vi "Start Sync.vi"(8 "error in (no error)":errorcluster, 11 "gRPC service in":refnum<class "OOBgRPCService.lvclass">) -> (0 "error out":errorcluster, 3 "gRPC service out":refnum<class "OOBgRPCService.lvclass">)   [LabVIEW 2025, in "OOB gRPC Server.lvlib" / "OOBgRPCService.lvclass"]
uses:
  OOBgRPCService.lvclass
  OOBgRPCService.lvclass/OOBgRPCService.ctl
  RPC Messages/hwval_GenericResponse.ctl
  RPC Messages/hwval_StatusResponse.ctl
  Buffer/Dequeue Frame.vi
  OOB Data Transfer/OOB Data Transfer.lvlib
  OOB gRPC Server.lvlib
  Automotive Ethernet Bus Monitor.lvclass
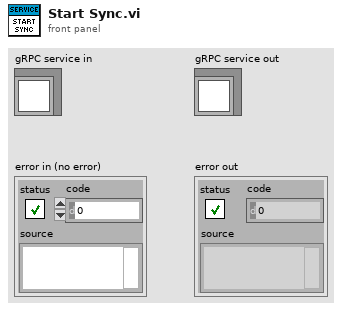
[diagram p1: front panel]
types:
  T1 = typedef "OOB gRPC Server.lvlib/hwval_GenericResponse.ctl" = cluster{"Payload":u8[]}
  T2 = typedef "OOB gRPC Server.lvlib/hwval_StatusResponse.ctl" = cluster{"Status":bool, "Code":i32, "Message":string}
  T3 = typedef "OOB gRPC Server.lvlib/OOBgRPCService.lvclass/Server Internal UEs.ctl" = cluster{"OOBgRPCService Generic Internal UE":refnum<user-event>, "OOBgRPCService PauseResume Internal UE":refnum<user-event>, "OOBgRPCService Export Internal UE":refnum<user-event>}
  T4 = typedef "OOB gRPC Server.lvlib/OOBgRPCService.lvclass/Server gRPC UEs.ctl" = cluster{"OOBgRPCService Generic gRPC UE":refnum<user-event>, "OOBgRPCService PauseResume gRPC UE":refnum<user-event>, "OOBgRPCService Export gRPC UE":refnum<user-event>}
  T5 = typedef "grpc-lvsupport-release.lvlib/grpcId.ctl" = u64
  T6 = typedef "OOB gRPC Server.lvlib/hwval_GenericRequest.ctl" = cluster{"Command":string, "Payload":u8[]}
  T7 = typedef "OOB Data Transfer.lvlib/OOB to Logic Data.ctl" = cluster{"PauseResume":bool, "Export":string}
  T8 = typedef "OOB gRPC Server.lvlib/hwval_BoolRequest.ctl" = cluster{"BooleanData":bool}
  T9 = typedef "OOB gRPC Server.lvlib/hwval_ExportRequest.ctl" = cluster{"FileType":string}
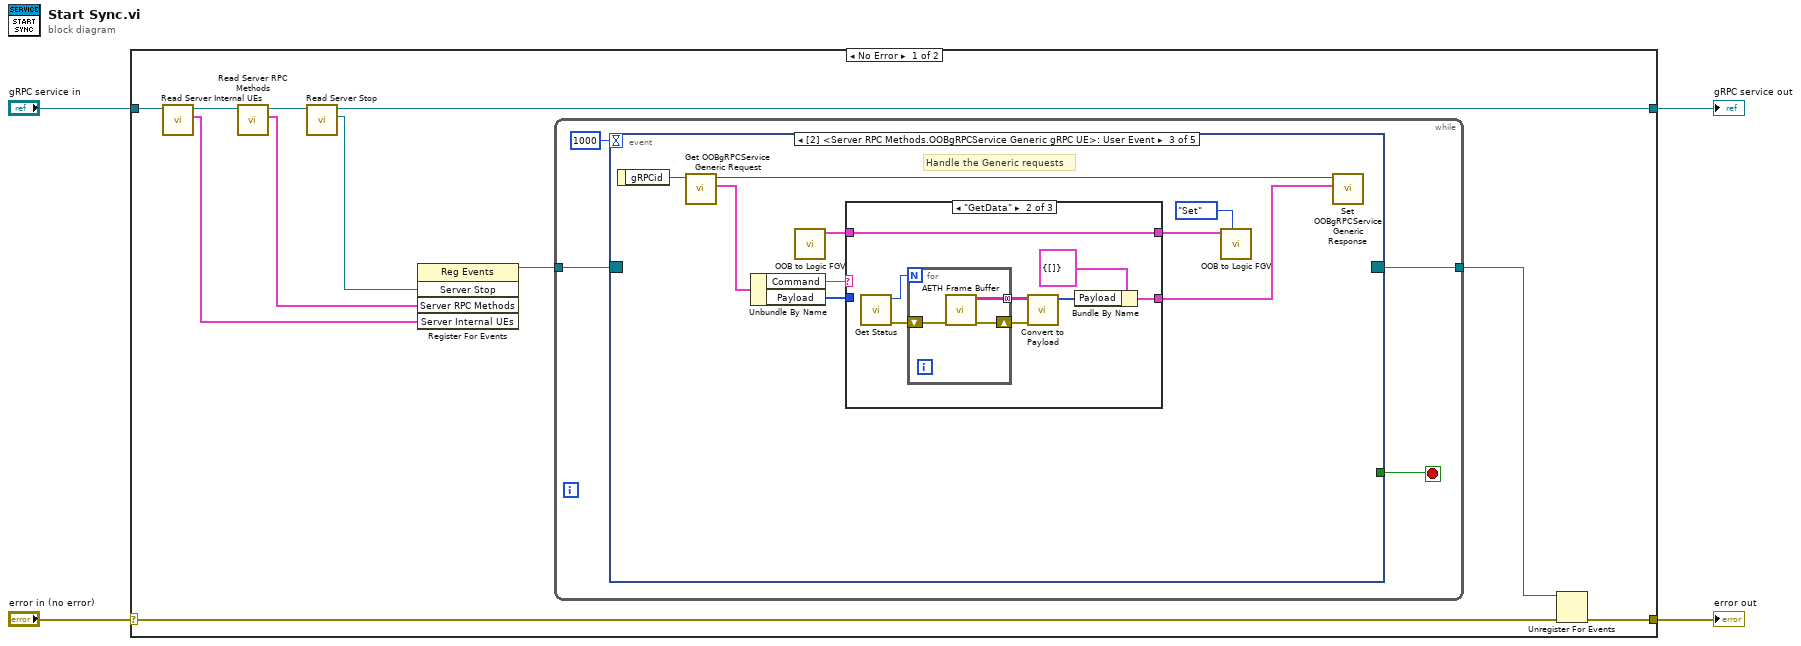
[diagram p0: block diagram]
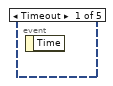
[diagram p2: hidden frame]
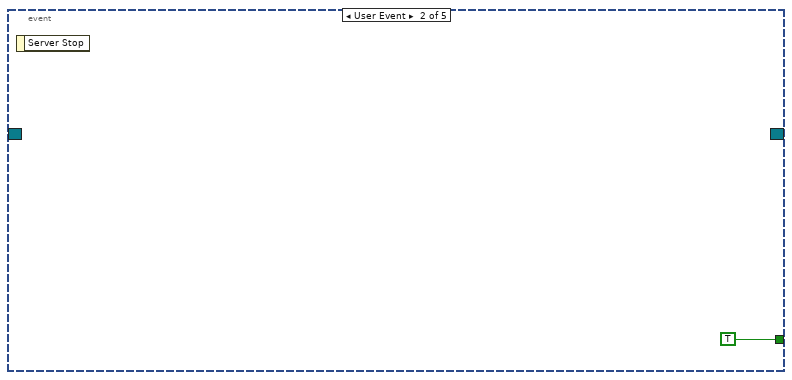
[diagram p3: hidden frame]
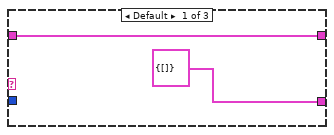
[diagram p4: hidden frame]
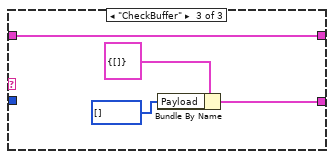
[diagram p5: hidden frame]
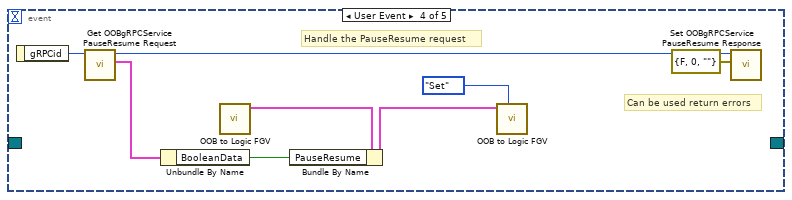
[diagram p6: hidden frame]
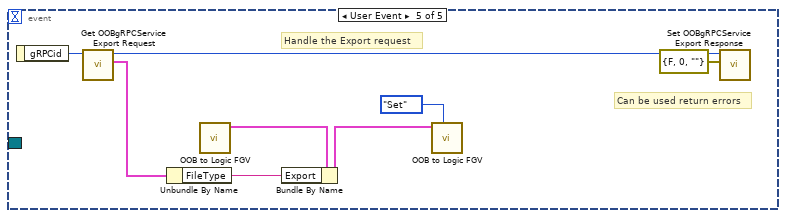
[diagram p7: hidden frame]
diagram:
  n1 = case shown="No Error" "error in (no error)" {
    selector: "error in (no error)" -> [w9 w64]
    tunnel: [w8 w64] -> w3
    tunnel: [w6 w63] -> w1
    tunnel: "gRPC service in" -> [w15 w63]
    frame No Error {
      n2 = call "Read Server Internal UEs.vi"("gRPC service in"=w15) -> ("Server Internal UEs"=w13:T3, "gRPC service out"=w14:refnum<class "OOBgRPCService.lvclass">)  [unwired: 8 in, 1 out]
      n3 = call "Read Server RPC Methods.vi"("gRPC service in"=w14) -> ("Server RPC Methods"=w7:T4, "gRPC service out"=w12:refnum<class "OOBgRPCService.lvclass">)  [unwired: 8 in, 1 out]
      n4 = call-dynamic "Read Server Stop.vi"("gRPC service in"=w12) -> ("Server Stop"=w5:refnum<user-event>, "gRPC service out"=w6:refnum<class "OOBgRPCService.lvclass">)  [unwired: 8 in, 1 out]
      n5 = register-events(w5, w7, w13) -> (reference out=w11:refnum<event-registration>)  [unwired: 2 in, 1 out]
      n6 = while {
        tunnel: w11 -> [w19]
        tunnel: [w17] -> w10
        stop <- w18 stop-if-true
        n7 = event "RPC Methods Event Structure" shown="[2] <Server RPC Methods.OOBgRPCService Generic gRPC UE>: User Event" {
          selector: w19 -> [_ _ _ _ _]
          dyn-events: [_ _ _ _ _] -> w17
          timeout: 1000 -> [_ _ _ _ _]
          tunnel: [_ TRUE _ _ _] -> w18
          event Timeout {
            n8 = event-data() -> ()  [unwired: 1 in, 1 out]
          }
          event User Event {
            n9 = event-data() -> ()  [unwired: 1 in, 1 out]
          }
          event User Event {
            # "Handle the Generic requests"
            n10 = event-data() -> ("gRPCid"=w29:T5)  [unwired: 1 in]
            n11 = call "Get OOBgRPCService Generic Request.vi"("gRPCid"=w29) -> ("Message Data"=w27:T6, "gRPCid out"=w28:T5)  [unwired: 8 in, 1 out]
            n12 = Unbundle By Name(w27) -> ("Command"=w23:string, "Payload"=w22:u8[])
            n13 = call "OOB to Logic FGV.vi"() -> ("OOB to Logic Data out"=w25:T7)  [unwired: 10 in, 1 out]
            n14 = case shown="\"GetData\"" w23 {
              tunnel: w25 -> [w31 w38 w46]
              tunnel: [w31 w38 w46] -> w24
              tunnel: w22 -> [_ _ _]
              tunnel: [T1 {"Payload"=[]} ("Message Data") w34 w44] -> w21
              frame Default {
              }
              frame "GetData" {
                n15 = call "Get Status.vi"() -> ("error out"=w33:errorcluster, "Messages"=w32:i32)  [unwired: 10 in]
                n16 = for {
                  N: w32 -> [_]
                  tunnel: [w41] -> w36 mode=concatenating
                  shift-right: [w42] -> w37
                  shift-left: w33 -> [w40]
                  n17 = call-poly "AETH Frame Buffer.vi"("error in"=w40) -> ("error out"=w42:errorcluster, "Data"=w41:string[][])  [unwired: 9 in]
                }
                n18 = call "Convert to Payload.vi"("error in"=w37, "Data"=w36) -> ("U8 Array"=w35:u8[])  [unwired: 8 in, 1 out]
                n19 = Bundle By Name(cluster=T1 {"Payload"=[]} ("Message Data"), "Payload"=w35) -> (w34:T1)
              }
              frame "CheckBuffer" {
                n20 = Bundle By Name(cluster=T1 {"Payload"=[]} ("Message Data"), "Payload"=u8[] []) -> (w44:T1)
              }
            }
            n21 = call "OOB to Logic FGV.vi"("Op (Get)"=enum16{"Get", "Set"}."Set", "OOB to Logic Data in"=w24) -> ()  [unwired: 8 in, 2 out]
            n22 = call "Set OOBgRPCService Generic Response.vi"("Message Data"=w21, "gRPCid in"=w28) -> ()  [unwired: 9 in, 1 out]
          }
          event User Event {
            # "Handle the PauseResume request"
            # "Can be used return errors"
            n23 = event-data() -> ("gRPCid"=w48:T5)  [unwired: 1 in]
            n24 = call "Get OOBgRPCService PauseResume Request.vi"("gRPCid"=w48) -> ("Message Data"=w50:T8, "gRPCid out"=w51:T5)  [unwired: 8 in, 1 out]
            n25 = Unbundle By Name(w50) -> ("BooleanData"=w49:bool)
            n26 = call "OOB to Logic FGV.vi"() -> ("OOB to Logic Data out"=w53:T7)  [unwired: 10 in, 1 out]
            n27 = Bundle By Name(cluster=w53, "PauseResume"=w49) -> (w52:T7)
            n28 = call "OOB to Logic FGV.vi"("Op (Get)"=enum16{"Get", "Set"}."Set", "OOB to Logic Data in"=w52) -> ()  [unwired: 8 in, 2 out]
            n29 = call "Set OOBgRPCService PauseResume Response.vi"("Message Data"=T2 {"Status"=FALSE, "Code"=0, "Message"=""}, "gRPCid in"=w51) -> ()  [unwired: 9 in, 1 out]
          }
          event User Event {
            # "Handle the Export request"
            # "Can be used return errors"
            n30 = event-data() -> ("gRPCid"=w56:T5)  [unwired: 1 in]
            n31 = call "Get OOBgRPCService Export Request.vi"("gRPCid"=w56) -> ("Message Data"=w58:T9, "gRPCid out"=w62:T5)  [unwired: 8 in, 1 out]
            n32 = Unbundle By Name(w58) -> ("FileType"=w57:string)
            n33 = call "OOB to Logic FGV.vi"() -> ("OOB to Logic Data out"=w60:T7)  [unwired: 10 in, 1 out]
            n34 = Bundle By Name(cluster=w60, "Export"=w57) -> (w59:T7)
            n35 = call "OOB to Logic FGV.vi"("Op (Get)"=enum16{"Get", "Set"}."Set", "OOB to Logic Data in"=w59) -> ()  [unwired: 8 in, 2 out]
            n36 = call "Set OOBgRPCService Export Response.vi"("Message Data"=T2 {"Status"=FALSE, "Code"=0, "Message"=""}, "gRPCid in"=w62) -> ()  [unwired: 9 in, 1 out]
          }
        }
      }
      n37 = Unregister For Events(event registration refnum=w10, error in=w9) -> (error out=w8:errorcluster)
    }
    frame Error {
    }
  }
  "error out" <- w3
  "gRPC service out" <- w1
